vi "Server Main.vi"() -> ()   [LabVIEW 2013]
doc: "WebSocket chat demo for sending/receiving chat messages with a web browser. Also a reasonable example of a multiple client TCP/IP architecture with launching VIs asynchronously for the lifetime of the connection."
uses:
  <vilib>/Intelligent Energy/Message Queue Helper/ctl_QMH_Message_Typedef.ctl
  WebSocket Server/ctl_Configuration.ctl
  Connection Handler/ctl_Message.ctl
  Connection Handler/ctl_ClientState.ctl
  <vilib>/Platform/browser.llb/Open URL in Default Browser (path).vi
  WebSocket Server/WebSocket Server.lvlib
  <vilib>/Intelligent Energy/Message Queue Helper/MessageQueueHelper.lvlib
  Connection Handler/Connection Handler.lvlib
panel:
  in  "Tab Control":enum32{"Server Console", "Embedded Client"}(tab)
  in  "Users":i32(listbox)
  in  "Message":string
  in  "Send":bool
  in  "Clear":bool
  out "Console":string
  in  "Open":bool
  in  "WebBrowser":refnum<k7>(container)
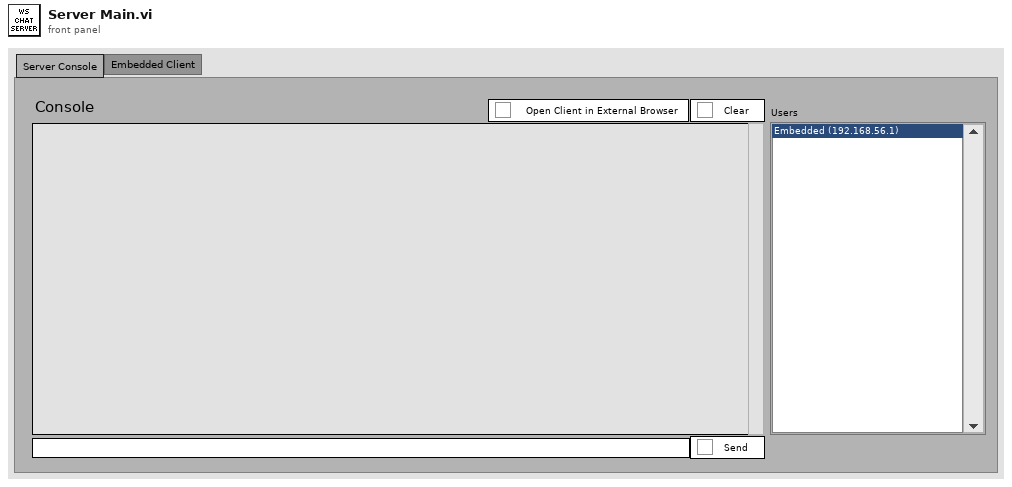
[diagram p1: front panel]
types:
  T1 = typedef "WebSocket Server.lvlib/ctl_Configuration.ctl" = cluster{"Listen Port":u16, "Handler Ref":refnum<vi>}
  T2 = typedef "MessageQueueHelper.lvlib/ctl_QMH_Message_Typedef.ctl" = cluster{"Command":string, "Data":variant}
  T3 = typedef "Connection Handler.lvlib/ctl_Message.ctl" = cluster{"username":string, "message":string}
  T4 = typedef "Connection Handler.lvlib/ctl_ClientState.ctl" = cluster{"Conn Ref":refnum<k5>, "IP Address":string, "Hostname":string, "User":cluster{"Username":string, "Read":bool, "Write":bool}}
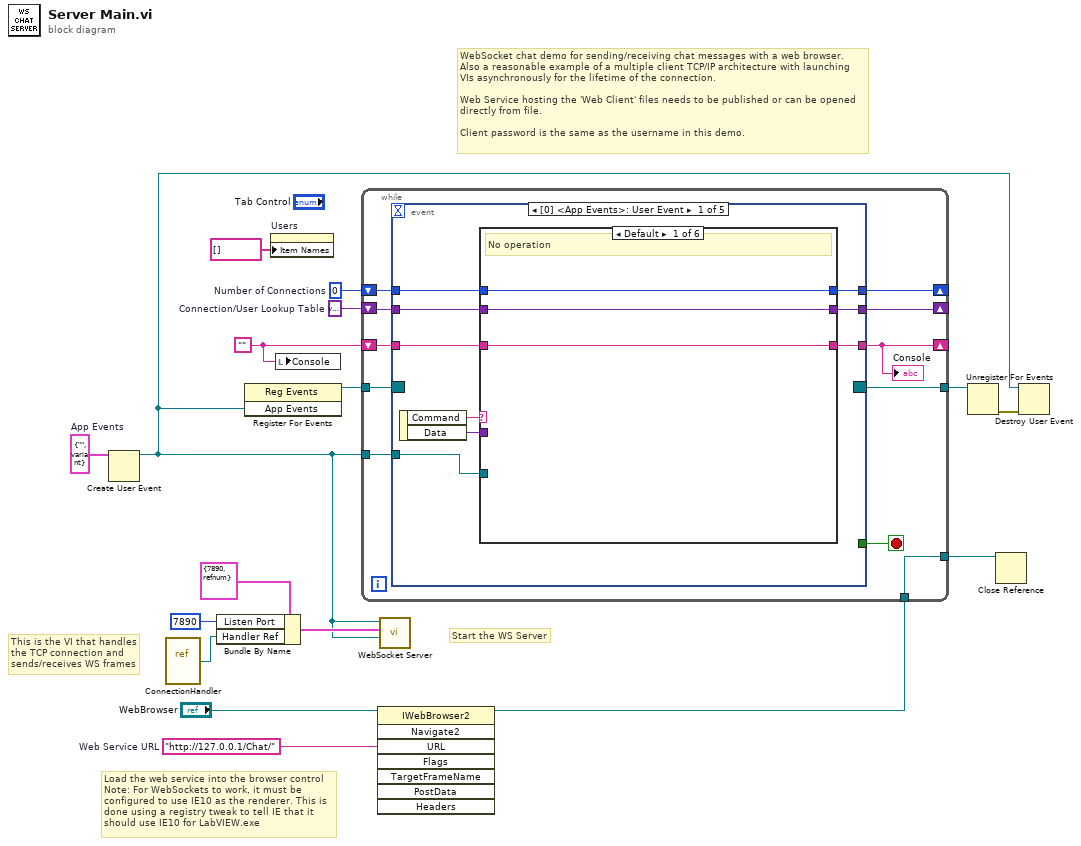
[diagram p0: block diagram]
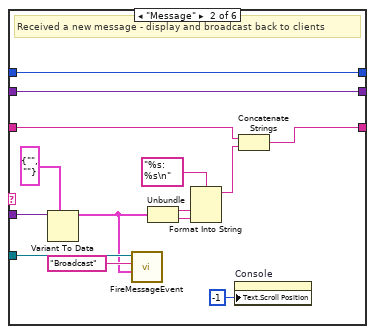
[diagram p2: hidden frame]
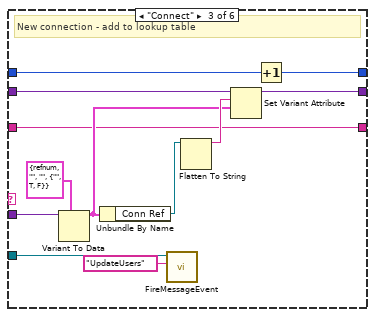
[diagram p3: hidden frame]
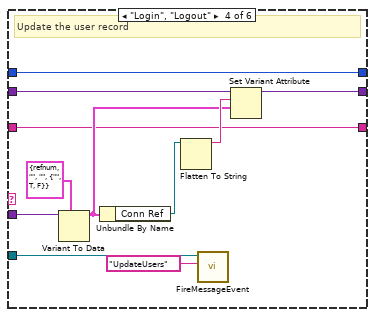
[diagram p4: hidden frame]
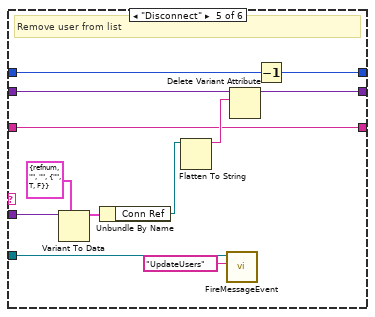
[diagram p5: hidden frame]
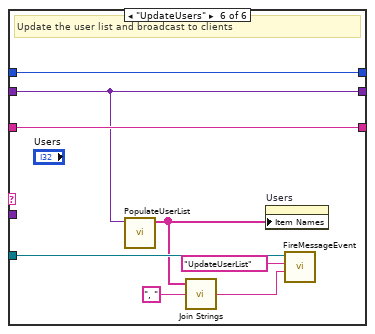
[diagram p6: hidden frame]
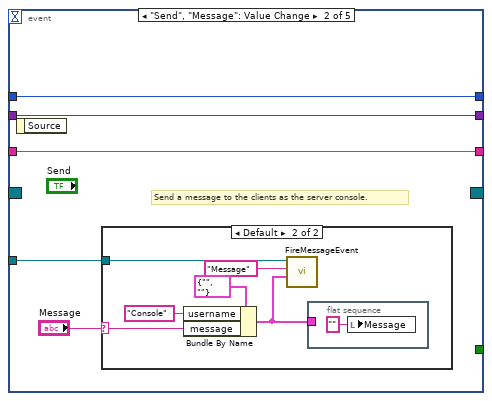
[diagram p7: hidden frame]
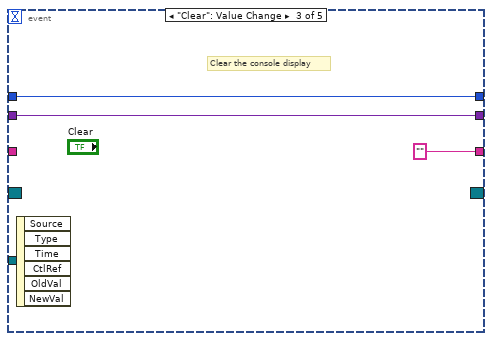
[diagram p9: hidden frame]
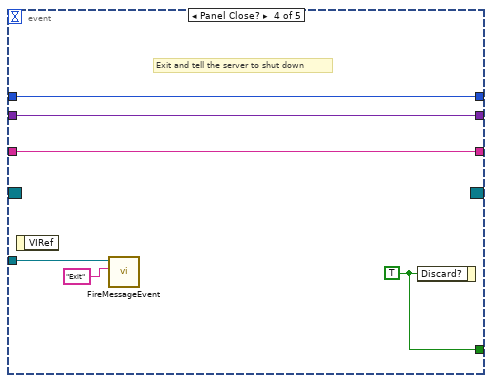
[diagram p10: hidden frame]
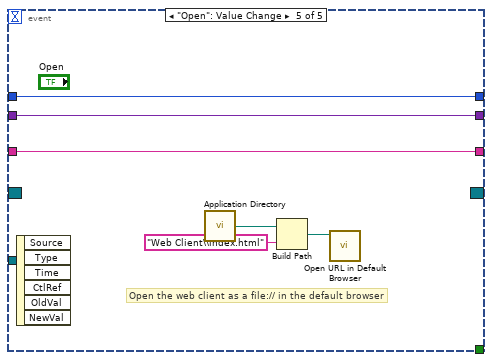
[diagram p11: hidden frame]
diagram:
  w4 = variant  # Connection/User Lookup Table
  w7 = "http://127.0.0.1/Chat/"  # Web Service URL
  w10 = 0  # Number of Connections
  w9 = ""
  w17 = T2 {"Command"="", "Data"=variant}  # App Events
  # "This is the VI that handles\nthe TCP connection and\nsends/receives WS frames"
  # "WebSocket chat demo for sending/receiving chat messages with a web browser. Also a reasonable example of a multiple client TCP/IP architecture with launching VIs asynchronously for the lifetime of the connection.\n\nWeb Service hosting the 'Web Client' files needs to be published or can be opened directly from file.\n\nClient password is the same as the username in this demo."
  # "Start the WS Server"
  # "Load the web service into the browser control\nNote: For WebSockets to work, it must be configured to use IE10 as the renderer. This is done using a registry tweak to tell IE that it should use IE10 for LabVIEW.exe"
  n1 = Create User Event(user event datatype=w17) -> (user event=w1:refnum<user-event>)  [unwired: 1 in, 1 out]
  n2 = vi-ref "ConnectionHandler.vi"() -> (w13:refnum<vi>)
  n3 = Bundle By Name(cluster=T1 {"Listen Port"=7890, "Handler Ref"=refnum} ("Configuration"), "Listen Port"=u16 7890, "Handler Ref"=w13) -> (w15:T1)
  n4 = register-events(w1) -> (reference out=w12:refnum<event-registration>)  [unwired: 2 in, 1 out]
  n5 = property on="Users" class="LstBox (strict)"("Item Names"=string[] []) -> ()  [unwired: 2 in, 2 out]
  n6 = local write "Console"(w9) -> ()
  n7 = invoke class="IWebBrowser2" method="Navigate2"(reference="WebBrowser", "URL"=w7) -> (reference out=w5:refnum<k7>)  [unwired: 6 in, 7 out]
  n8 = while {
    tunnel: w1 -> [w27]
    tunnel: w12 -> [w26]
    tunnel: [w25] -> w11
    shift-right: [w24] -> _
    shift-left: w9 -> [w21]
    shift-right: [w22] -> _
    shift-left: w10 -> [w23]
    tunnel: w5 -> [w20]
    tunnel: [w20] -> w6
    shift-right: [w18] -> _
    shift-left: w4 -> [w19]
    stop <- w28 stop-if-true
    n9 = event shown="[0] <App Events>: User Event" {
      selector: w26 -> [_ _ _ _ _]
      dyn-events: [_ _ _ _ _] -> w25
      timeout: _ -> [_ _ _ _ _]
      tunnel: [_ _ _ w118 _] -> w28
      tunnel: w27 -> [w33 w101 _ w117 _]
      tunnel: [w35 w102 "" w115 w124] -> w24
      tunnel: w21 -> [w34 w102 _ w115 w124]
      tunnel: w23 -> [w32 w99 w111 w114 w123]
      tunnel: [w31 w99 w111 w114 w123] -> w22
      tunnel: w19 -> [w30 w98 w110 w113 w119]
      tunnel: [w29 w98 w110 w113 w119] -> w18
      event User Event {
        n10 = event-data() -> ("Command"=w37:string, "Data"=w36:variant)  [unwired: 1 in]
        n11 = case shown="Default" w37 {
          tunnel: w36 -> [_ w54 w64 w76 w87 _]
          tunnel: [w40 w48 w57 w69 w80 w97] -> w35
          tunnel: w34 -> [w40 w47 w57 w69 w80 w97]
          tunnel: w33 -> [_ w46 w56 w67 w78 w94]
          tunnel: w32 -> [w39 w43 w66 w77 w89 w96]
          tunnel: [w39 w43 w65 w77 w88 w96] -> w31
          tunnel: w30 -> [w38 w41 w62 w74 w82 w95]
          tunnel: [w38 w41 w61 w73 w83 w95] -> w29
          frame Default {
            # "No operation"
          }
          frame "Message" {
            # "Received a new message - display and broadcast back to clients"
            n12 = Variant To Data(type=T3 {"username"="", "message"=""}, Variant=w54) -> (data=w44:T3)  [unwired: 1 in, 1 out]
            n13 = call <vilib>:"FireMessageEvent.vi"("Data"=w44, "Command"="Broadcast", "User Event in"=w46) -> ()  [unwired: 7 in, 2 out]
            n14 = Unbundle(w44) -> ("username"=w51:string, "message"=w50:string)
            n15 = Format Into String(format string="%s: %s\n", w51, w50) -> (resulting string=w49:string)  [unwired: 2 in, 1 out]
            n16 = property on="Console" class="Str"("Text.Scroll Position"=-1) -> ()  [unwired: 2 in, 2 out]
            n17 = Concatenate Strings(w47, w49) -> (w48:string)
          }
          frame "Connect" {
            # "New connection - add to lookup table"
            n18 = Variant To Data(type=T4 {"Conn Ref"=refnum, "IP Address"="", "Hostname"="", "User"={"Username"="", "Read"=TRUE, "Write"=FALSE}} ("State out"), Variant=w64) -> (data=w58:T4)  [unwired: 1 in, 1 out]
            n19 = Unbundle By Name(w58) -> ("Conn Ref"=w59:refnum<k5>)
            n20 = call <vilib>:"FireMessageEvent.vi"("Command"="UpdateUsers", "User Event in"=w56) -> ()  [unwired: 8 in, 2 out]
            n21 = Flatten To String(anything=w59) -> (data string=w60:string)  [unwired: 3 in, 2 out]
            n22 = Set Variant Attribute(Variant=w62, name=w60, value=w58) -> (Variant out=w61:variant)  [unwired: 1 in, 2 out]
            n23 = Increment(x=w66) -> (x+1=w65:i32)
          }
          frame "Login", "Logout" {
            # "Update the user record"
            n24 = Variant To Data(type=T4 {"Conn Ref"=refnum, "IP Address"="", "Hostname"="", "User"={"Username"="", "Read"=TRUE, "Write"=FALSE}} ("State out"), Variant=w76) -> (data=w70:T4)  [unwired: 1 in, 1 out]
            n25 = Unbundle By Name(w70) -> ("Conn Ref"=w71:refnum<k5>)
            n26 = Flatten To String(anything=w71) -> (data string=w72:string)  [unwired: 3 in, 2 out]
            n27 = call <vilib>:"FireMessageEvent.vi"("Command"="UpdateUsers", "User Event in"=w67) -> ()  [unwired: 8 in, 2 out]
            n28 = Set Variant Attribute(Variant=w74, name=w72, value=w70) -> (Variant out=w73:variant)  [unwired: 1 in, 2 out]
          }
          frame "Disconnect" {
            # "Remove user from list"
            n29 = Variant To Data(type=T4 {"Conn Ref"=refnum, "IP Address"="", "Hostname"="", "User"={"Username"="", "Read"=TRUE, "Write"=FALSE}} ("State out"), Variant=w87) -> (data=w84:T4)  [unwired: 1 in, 1 out]
            n30 = Unbundle By Name(w84) -> ("Conn Ref"=w85:refnum<k5>)
            n31 = Flatten To String(anything=w85) -> (data string=w81:string)  [unwired: 3 in, 2 out]
            n32 = call <vilib>:"FireMessageEvent.vi"("Command"="UpdateUsers", "User Event in"=w78) -> ()  [unwired: 8 in, 2 out]
            n33 = Delete Variant Attribute(6:w81, 7:w82) -> (3:w83:variant)  [unwired: 1 in, 2 out]
            n34 = Decrement(x=w89) -> (x-1=w88:i32)
          }
          frame "UpdateUsers" {
            # "Update the user list and broadcast to clients"
            n35 = call "PopulateUserList.vi"("Variant"=w95) -> ("Array"=w92:string[])  [unwired: 9 in, 1 out]
            n36 = call <vilib>:"Join Strings.vi"("Separator (,)"=", ", "Strings In"=w92) -> ("String"=w91:string)  [unwired: 1 in]
            n37 = property on="Users" class="LstBox (strict)"("Item Names"=w92) -> ()  [unwired: 2 in, 2 out]
            n38 = call <vilib>:"FireMessageEvent.vi"("Data"=w91, "Command"="UpdateUserList", "User Event in"=w94) -> ()  [unwired: 7 in, 2 out]
          }
        }
      }
      event "Send", "Message": Value Change {
        # "Send a message to the clients as the server console."
        n39 = event-data() -> ()  [unwired: 1 in, 1 out]
        n40 = case shown="Default" "Message" {
          selector: "Message" -> [_ w103]
          tunnel: w101 -> [_ w107]
          frame "" {
          }
          frame Default {
            n41 = Bundle By Name(cluster=T3 {"username"="", "message"=""}, "username"="Console", "message"=w103) -> (w104:T3)
            n42 = call <vilib>:"FireMessageEvent.vi"("Data"=w104, "Command"="Message", "User Event in"=w107) -> ()  [unwired: 7 in, 2 out]
            n43 = flat-sequence {
              tunnel: w104 -> [_]
              frame #0 {
                n44 = local write "Message"("" ("Message")) -> ()
              }
            }
          }
        }
      }
      event "Clear": Value Change {
        # "Clear the console display"
        n45 = event-data() -> ()  [unwired: 1 in, 6 out]
      }
      event Panel Close? {
        w118 = TRUE
        # "Exit and tell the server to shut down"
        n46 = event-data() -> ()  [unwired: 1 in, 1 out]
        n47 = call <vilib>:"FireMessageEvent.vi"("Command"="Exit", "User Event in"=w117) -> ()  [unwired: 8 in, 2 out]
        n48 = event-data("Discard?"=w118) -> ()  [unwired: 1 in, 1 out]
      }
      event "Open": Value Change {
        # "Open the web client as a file:// in the default browser"
        n49 = event-data() -> ()  [unwired: 1 in, 6 out]
        n50 = call <vilib>:"Application Directory.vi"() -> ("Application Directory"=w121:path)
        n51 = Build Path(base path=w121, name or relative path="Web Client\\index.html") -> (appended path=w122:path)
        n52 = call-poly <vilib>:"Open URL in Default Browser.vi"("path"=w122) -> ()  [unwired: 5 in, 2 out]
      }
    }
    "Console" <- w24
  }
  n53 = call "WebSocket Server.vi"("Handler References"=w1, "Configuration"=w15, "Main Event"=w1) -> ()  [unwired: 8 in, 1 out]
  n54 = Unregister For Events(event registration refnum=w11) -> (error out=w2:errorcluster)  [unwired: 1 in]
  n55 = Close Reference(reference=w6) -> ()  [unwired: 1 in, 1 out]
  n56 = Destroy User Event(user event=w1, error in=w2) -> ()  [unwired: 1 out]
